vi "Start Test For Candidate.vi"(10 "Candidate_ID":string, 11 "Candidates":T1[](array[typedef])) -> (3 "Candidates out":T1[](array[typedef]))   [LabVIEW 2014, in "Coding Platform.lvlib"]
uses:
  Coding Platform.lvlib
  Typedefs/Candidate.ctl
  Typedefs/Candidate State.ctl
  Typedefs/Answer Info.ctl
  Typedefs/Answer State.ctl
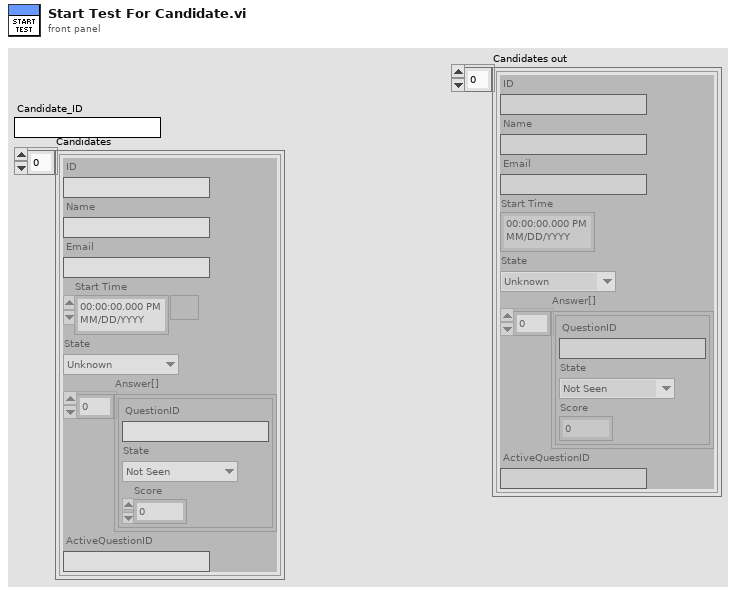
[diagram p1: front panel]
types:
  T1 = typedef "Coding Platform.lvlib/Candidate.ctl" = cluster{"ID":string, "Name":string, "Email":string, "Start Time":timestamp, "State":T2, "Answer[]":T3[], "ActiveQuestionID":string}
  T2 = typedef "Coding Platform.lvlib/Candidate State.ctl" = enum16{"Unknown", "LoggedIn", "In Test", "Completed Test"}
  T3 = typedef "Coding Platform.lvlib/Answer Info.ctl" = cluster{"QuestionID":string, "State":T4, "Score":u64}
  T4 = typedef "Coding Platform.lvlib/Answer State.ctl" = enum16{"Not Seen", "In Progress", "Completed"}
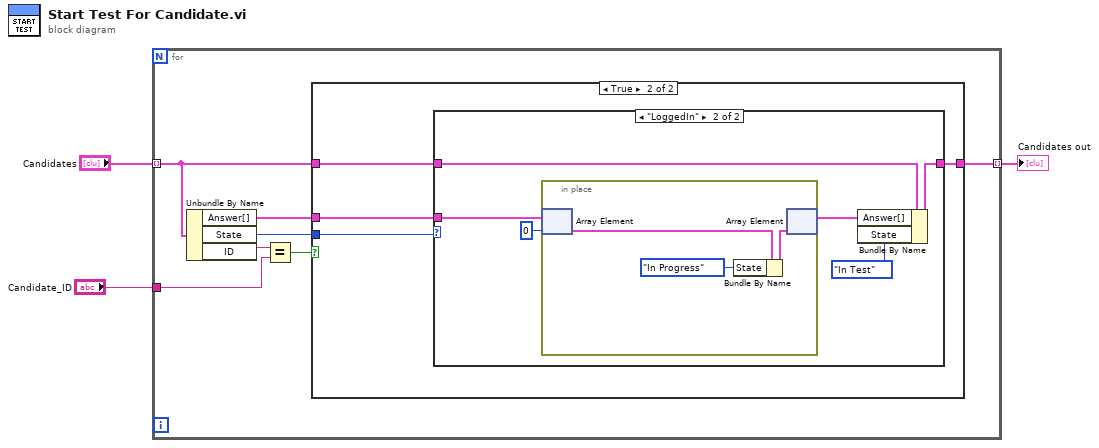
[diagram p0: block diagram]
diagram:
  n1 = for {
    tunnel: "Candidate_ID" -> [w9]
    tunnel: [w6] -> w1 mode=indexing
    tunnel: "Candidates" -> [w5] mode=indexing
    n2 = Unbundle By Name(w5) -> ("Answer[]"=w4:T3[], "State"=w7:T2, "ID"=w10:string)
    n3 = Equal?(x=w10, y=w9) -> (x = y?=w8:bool)
    n4 = case shown="True" w8 {
      tunnel: w7 -> [_ w12]
      tunnel: [w11 w13] -> w6
      tunnel: w5 -> [w11 w15]
      tunnel: w4 -> [_ w14]
      frame False {
      }
      frame True {
        n5 = case shown="\"LoggedIn\"" w12 {
          tunnel: w15 -> [w16 w22]
          tunnel: w14 -> [_ w21]
          tunnel: [w16 w20] -> w13
          frame "Unknown", Default {
          }
          frame "LoggedIn" {
            n6 = in-place {
              n7 = in-place-array #1(w21, 0) -> (w25:T3)
              n8 = Bundle By Name(cluster=w25, "State"=Answer_State."In Progress") -> (w24:T3)
              n9 = in-place-array #1(w24) -> (w19:T3[])  [unwired: 1 out]
            }
            n10 = Bundle By Name(cluster=w22, "Answer[]"=w19, "State"=Candidate_State."In Test") -> (w20:T1)
          }
        }
      }
    }
  }
  "Candidates out" <- w1
